vi "Save_Config.vi"() -> ()   [LabVIEW 2020]
uses:
  <vilib>/Platform/TimedLoop/XDataNode/timing_clust.ctl
  <vilib>/Platform/TimedLoop/XDataNode/nitl_modes.ctl
  <vilib>/Platform/TimedLoop/XDataNode/wakeup.ctl
  <vilib>/CANopenLib/CANOPEN.llb/CANopen Interface Create.vi
  <vilib>/CANopenLib/CANOPEN.llb/CANopen CAN Frame Read Create.vi
  <vilib>/CANopenLib/CANOPEN.llb/CANopen CAN Frame Read Start.vi
  <vilib>/CANopenLib/CANOPEN.llb/CANopen CAN Frame Read Close.vi
  <vilib>/CANopenLib/CANOPEN.llb/CANopen Interface Close.vi
  <vilib>/Platform/TimedLoop/XDataNode/XDataNode.xnode
  <vilib>/Platform/TimedLoop/XDataNode/XDNodeRunTimeDep.lvlib
panel:
  out "COB-ID":u32 format="%.0x"
  out "RTR?":bool
  out "timestamp":timestamp
  out "new data?":bool
  in  "stop":bool
  in  "RTR? (F)":bool
  in  "COB-ID (0)":u32=1539 format="%.0x"
  in  "CAN message data out":u8[](array[numeric])=[35, 16, 16, 1, 115, 97, 118, 101] format="%x"
  in  "write":bool
  out "CAN message data":u8[](array[numeric]) format="%x"
  in  "period (ms)":i64=10
  in  "buffer size (0)":u16=5
  in  "node-ID":u8=1 min=1 max=127 step=1
  in  "baud rate":u32(ring)=2 items=["1 Mbit/s"=0, "800 kbit/s"=1, "500 kbit/s"=2, "250 kbit/s"=3, "125 kbit/s"=4, "50 kbit/s"=6, "20 kbit/s"=7, "10 kbit/s"=8]
  in  "CANopen interface":u32(ring)=2 items=["CANopen01", "CANopen02", "CANopen03", "CANopen04", "CANopen05", "CANopen06", "CANopen07", "CANopen08", "CANopen09", "CANopen10", "CANopen11", "CANopen12", "CANopen13", "CANopen14", "CANopen15", "CANopen16", "CANopen17", "CANopen18", "CANopen19", "CANopen20", "CANopen21", "CANopen22", "CANopen23", "CANopen24", "CANopen25", "CANopen26", "CANopen27", "CANopen28", "CANopen29", "CANopen30", "CANopen31", "CANopen32"]
  # "保存参数 （修改前面的参数都必须执行保存参数，然后断电重启）\nCANID:601\nDATA: 23 10 10 01 73 61 76 65\n前面括号内为你需要修改的值\n\nwrite data项类型为u32\n最后需要关闭节点"
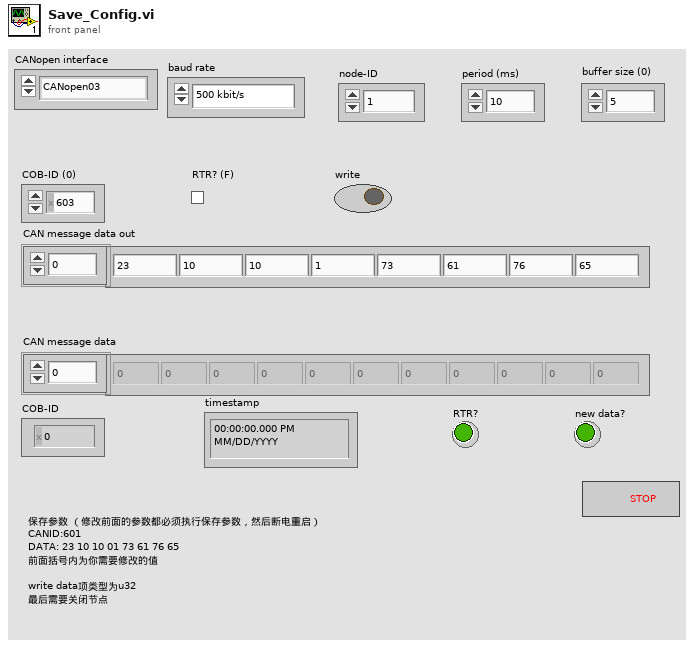
[diagram p1: front panel]
types:
  T1 = typedef "XDNodeRunTimeDep.lvlib/timing_clust.ctl" = cluster{"Expected End [f-1]":u64, "Actual End [f-1]":u64, "Finished Late? [f-1]":bool, "Expected End [i-1]":u64, "Actual End [i-1]":u64, "Finished Late? [i-1]":bool, "Expected Start [i]":u64, "Actual Start [i]":u64, "Expected Start [f]":u64, "Actual Start [f]":u64, "Source Name":string, "Structure Name":string, "Period":i64, "Deadline":i64, "Offset":i64, "Start":i64, "Priority":i32, "Timeout":i32, "Mode":T2, "Wakeup Reason":T3, "Error":errorcluster, "Source Type":string, "Secondary Source Type":string, "Global End Time":u64, "Global Start Time":u64, "Frame Duration":u64, "Iteration Duration":u64, "Assigned CPU":i32, "I/O Scan Engine Mode":u32}
  T2 = typedef "XDNodeRunTimeDep.lvlib/nitl_modes.ctl" = enum32{"No Change", "Process missed periods, maintain original phase", "Discard missed periods, maintain original phase", "Process missed periods, ignore original phase", "Discard missed periods, ignore original phase"}
  T3 = typedef "XDNodeRunTimeDep.lvlib/wakeup.ctl" = enum32{"Normal", "Aborted", "Asynchronous wakeup", "Timing source error", "Timed loop error", "Timeout"}
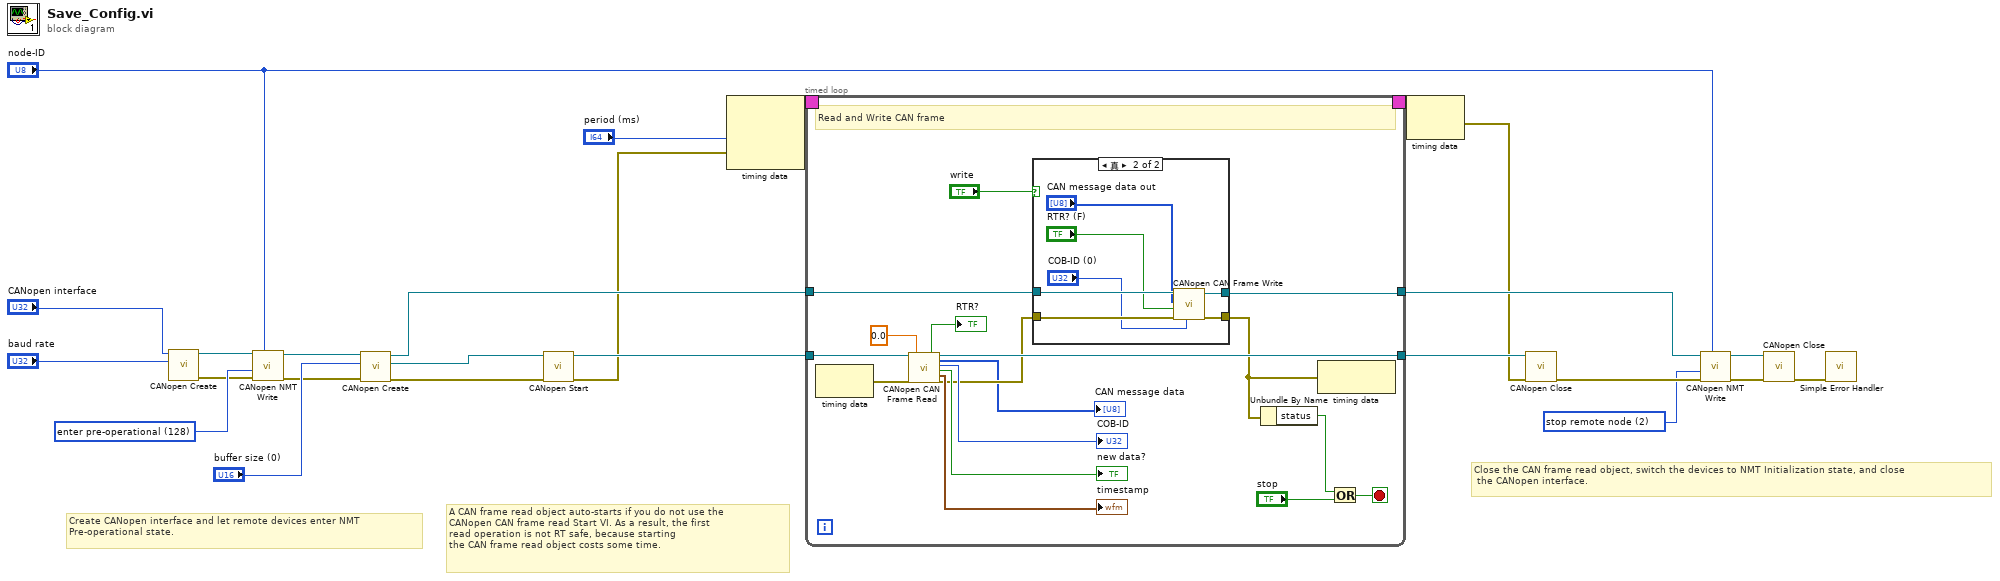
[diagram p0: block diagram]
diagram:
  w9 = u16 2 items=["start remote node"=1, "stop remote node"=2, "enter pre-operational"=128, "reset node"=129, "reset communication"=130] ("command")
  w21 = u16 128 items=["start remote node"=1, "stop remote node"=2, "enter pre-operational"=128, "reset node"=129, "reset communication"=130] ("command")
  # "A CAN frame read object auto-starts if you do not use the \nCANopen CAN frame read Start VI. As a result, the first \nread operation is not RT safe, because starting \nthe CAN frame read object costs some time."
  # "Close the CAN frame read object, switch the devices to NMT Initialization state, and close\n the CANopen interface."
  # "Create CANopen interface and let remote devices enter NMT\nPre-operational state."
  n1 = call-poly <vilib>:"CANopen Create.vi"("baud rate"="baud rate", "interface name"="CANopen interface") -> ("error out"=w20:errorcluster, "interface object out"=w19:refnum<k20>)  [unwired: 8 in]
  n2 = call <vilib>:"CANopen NMT Write.vi"("node-ID (0)"="node-ID", "error in (no error)"=w20, "command"=w21, "interface object in"=w19) -> ("error out"=w16:errorcluster, "interface object out"=w15:refnum<k20>)  [unwired: 6 in]
  n3 = call-poly <vilib>:"CANopen Create.vi"("error in (no error)"=w16, "buffer size (0)"="buffer size (0)", "interface object in"=w15) -> ("error out"=w6:errorcluster, "CAN frame read object out"=w8:refnum<k20>, "interface object out"=w7:refnum<k20>)  [unwired: 6 in]
  n4 = call-poly <vilib>:"CANopen Start.vi"("error in (no error)"=w6, "CAN frame read object in"=w8) -> ("error out"=w4:errorcluster, "CAN frame read object out"=w14:refnum<k20>)  [unwired: 8 in]
  n5 = node-c288("period (ms)", w4) -> (w25:T1)  [unwired: 1 in]
  n6 = timed-loop {
    tunnel: w14 -> [w27]
    tunnel: [w42] -> w17
    tunnel: w7 -> [w33]
    tunnel: [w34] -> w13
    timing: w25 -> [_]
    timing-out: [_] -> w24
    stop <- w36 stop-if-true
    # "Read and Write CAN frame"
    n7 = node-c288() -> (w30:errorcluster)  [unwired: 1 in]
    n8 = call <vilib>:"CANopen CAN Frame Read.vi"("CAN frame read object in"=w27, "error in (no error)"=w30, "timeout (0s)"=0.0 ("timeout(0)")) -> ("RTR?"=→"RTR?":bool, "CAN frame read object out"=w42:refnum<k20>, "CAN message data"=→"CAN message data":u8[], "COB-ID"=→"COB-ID":u32, "new data?"=→"new data?":bool, "timestamp"=→"timestamp":timestamp, "error out"=w32:errorcluster)  [unwired: 10 in]
    n9 = case shown="真" "write" {
      tunnel: [w49 w56] -> w34
      tunnel: w33 -> [w49 w55]
      tunnel: w32 -> [w48 w54]
      tunnel: [w48 w53] -> w29
      frame False {
      }
      frame True {
        n10 = call <vilib>:"CANopen CAN Frame Write.vi"("COB-ID (0)"="COB-ID (0)", "error in (no error)"=w54, "RTR? (F)"="RTR? (F)", "CAN message data"="CAN message data out", "interface object  in"=w55) -> ("error out"=w53:errorcluster, "interface object out"=w56:refnum<k20>)  [unwired: 5 in]
      }
    }
    n11 = Unbundle By Name(w29) -> ("status"=w35:bool)
    n12 = node-c288(w29) -> ()  [unwired: 1 out]
    n13 = Or(x=w35, y="stop") -> (x .or. y?=w36:bool)
  }
  n14 = node-c288(w24) -> (w3:errorcluster)
  n15 = call-poly <vilib>:"CANopen Close.vi"("error in (no error)"=w3, "CAN frame read object in"=w17) -> ("error out"=w11:errorcluster)  [unwired: 9 in]
  n16 = call <vilib>:"CANopen NMT Write.vi"("node-ID (0)"="node-ID", "error in (no error)"=w11, "command"=w9, "interface object in"=w13) -> ("error out"=w10:errorcluster, "interface object out"=w12:refnum<k20>)  [unwired: 6 in]
  n17 = call-poly <vilib>:"CANopen Close.vi"("error in (no error)"=w10, "interface object in"=w12) -> ("error out"=w1:errorcluster)  [unwired: 9 in]
  n18 = call <vilib>:"Simple Error Handler.vi"("error in (no error)"=w1) -> ()  [unwired: 4 in, 5 out]
